vi "Acquisition & Generation (Init Memory) test.vi"   [LabVIEW 2014]
uses:
  <vilib>/Platform/TimedLoop/XDataNode/timing_clust.ctl
  <vilib>/Platform/TimedLoop/XDataNode/nitl_modes.ctl
  <vilib>/Platform/TimedLoop/XDataNode/wakeup.ctl
  <vilib>/rvi/Emulation/niFpgaSctlEmulationGetInTimedLoop.vi
  <vilib>/rvi/Emulation/niFpgaEmulationReportErrorSimple.vi
  <vilib>/rvi/Emulation/niFpgaGetClockAttributes.vi
  <vilib>/rvi/Emulation/niFpgaCriticalErrorInLSC.vi
  <vilib>/rvi/Memory/Memory_Emulation/nirvimemoryFastEmulation.vi
  <vilib>/rvi/Memory/Memory_Emulation/nirvimemoryEmulation.vi
  <vilib>/rvi/Emulation/niFpgaEmulationIsFPGAContextNoSignature.vi
  <vilib>/rvi/DataTransferAndStorage/Container/Common/niFpgaContainerGetUniqueNameForEmu.vi
  <vilib>/rvi/Emulation/niFpgaProcessEmulError.vi
  <vilib>/rvi/errors/nirviReportUnexpectedCaseInternalError (U32).vi
  <vilib>/rvi/errors/niFpgaSetErrorForExecOnDevCompSimple.vi
  <vilib>/rvi/eio/common/nirviEmuReportErrorAndStop.vi
  <vilib>/rvi/FIFO/Fifo_Resource/nirvififoEmulationSetSize.vi
  <vilib>/rvi/FIFO/Fifo_Resource/nirviFifoEmulationQueueMgr.vi
  <instcachedir>/0/nirviFifoEmulationQueueMgr_E5CAEC123FF24DC58D834DCA3CDAA9B5.lvgen/nirviFifoEmulationQueueMgr_E5CAEC123FF24DC58D834DCA3CDAA9B5_010.vi
  <vilib>/rvi/FIFO/Fifo_Resource/nirvififoEmulationDetermineInputValidOut.vi
  <vilib>/rvi/FIFO/Fifo_Resource/nirvififoEmulationCreateLock.vi
  <vilib>/rvi/FIFO/Fifo_Resource/nirvififoEmulationObtainLock.vi
  <vilib>/rvi/FIFO/Fifo_Resource/nirvififoEmulationReleaseLock.vi
  <vilib>/rvi/occurrence/nirviWaitOnOccurrenceBase.vi
  <vilib>/rvi/errors/nirviReportUnexpectedCaseInternalError.vi
  <vilib>/rvi/interface/RandomDataEmulation/niFpgaRandomDataHandleErrors.vi
  <vilib>/rvi/eio/common/nirviEmuTemplateMethod_errors.vi
  <vilib>/Platform/TimedLoop/XDataNode/XDataNode.xnode
  <vilib>/rvi/DataTransferAndStorage/Container/XNode/niFpgaContainer.xnode
  <vilib>/rvi/FIFO/Fifo_Resource/nirvififoEmulationWrite.vi
  <vilib>/rvi/interface/RandomDataEmulation/nirviRandomDataFpgaReadWriteTemplate.vi
  <vilib>/rvi/FIFO/Fifo_Resource/nirvififoEmulationRead.vi
  <vilib>/eio/EIOMethodNode/EIOMethodNode.xnode
  <vilib>/Platform/TimedLoop/XDataNode/XDNodeRunTimeDep.lvlib
types:
  T1 = typedef "XDNodeRunTimeDep.lvlib/timing_clust.ctl" = cluster{"Expected End [f-1]":u64, "Actual End [f-1]":u64, "Finished Late? [f-1]":bool, "Expected End [i-1]":u64, "Actual End [i-1]":u64, "Finished Late? [i-1]":bool, "Expected Start [i]":u64, "Actual Start [i]":u64, "Expected Start [f]":u64, "Actual Start [f]":u64, "Source Name":string, "Structure Name":string, "Period":i64, "Deadline":i64, "Offset":i64, "Start":i64, "Priority":i32, "Timeout":i32, "Mode":T2, "Wakeup Reason":T3, "Error":errorcluster, "Source Type":string, "Secondary Source Type":string, "Global End Time":u64, "Global Start Time":u64, "Frame Duration":u64, "Iteration Duration":u64, "Assigned CPU":i32, "I/O Scan Engine Mode":u32}
  T2 = typedef "XDNodeRunTimeDep.lvlib/nitl_modes.ctl" = enum32{"No Change", "Process missed periods, maintain original phase", "Discard missed periods, maintain original phase", "Process missed periods, ignore original phase", "Discard missed periods, ignore original phase"}
  T3 = typedef "XDNodeRunTimeDep.lvlib/wakeup.ctl" = enum32{"Normal", "Aborted", "Asynchronous wakeup", "Timing source error", "Timed loop error", "Timeout"}
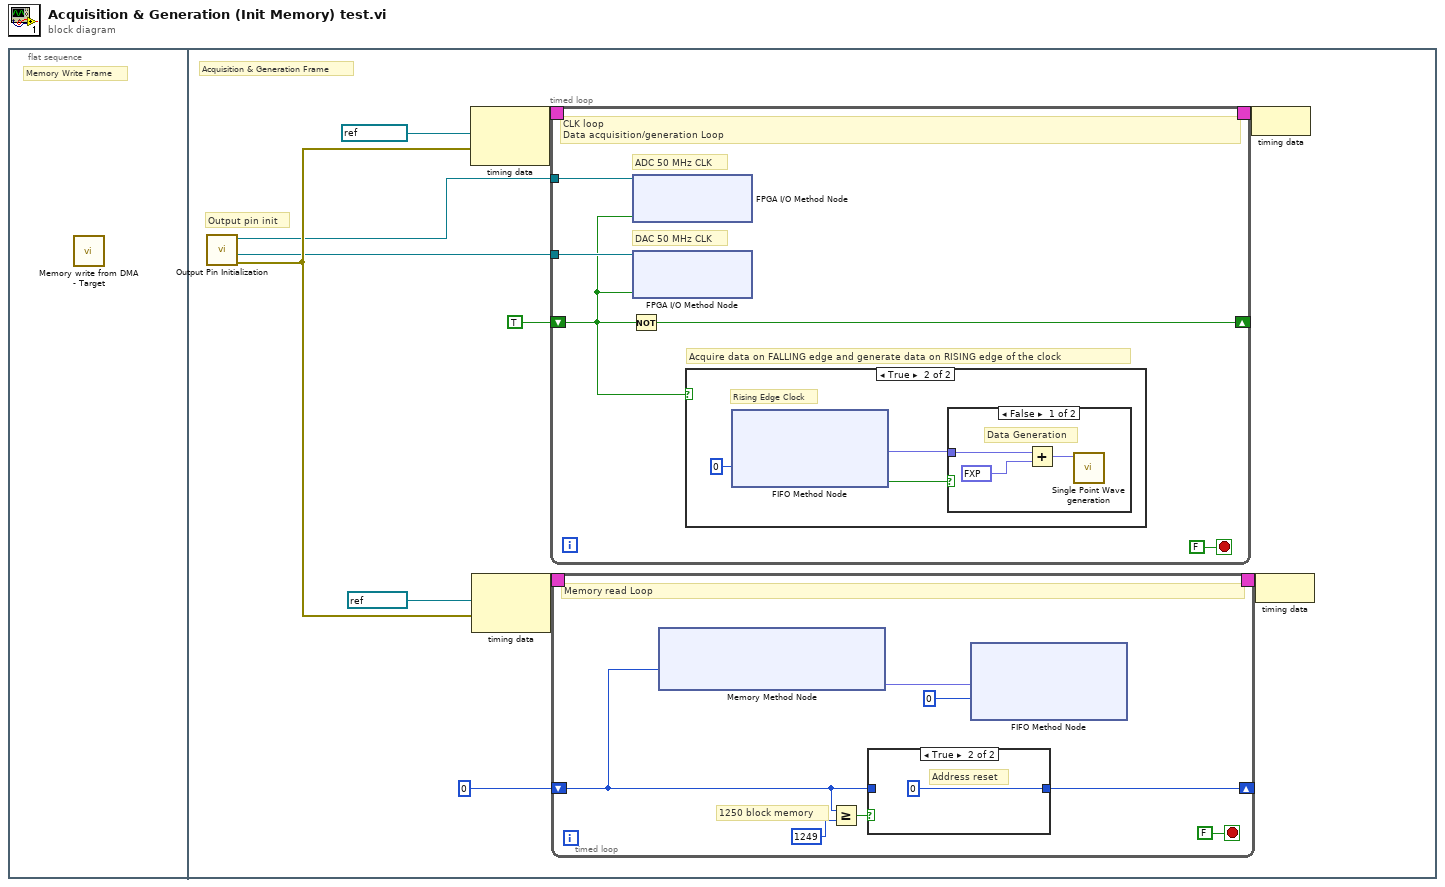
[diagram p0: block diagram]
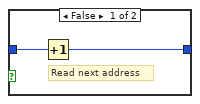
[diagram p2: hidden frame]
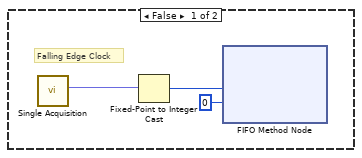
[diagram p3: hidden frame]
diagram:
  n1 = flat-sequence {
    frame #0 {
      # "Memory Write Frame"
      n2 = call "Memory write from DMA - Target.vi"() -> ()  [unwired: 12 in]
    }
    frame #1 {
      # "Acquisition & Generation Frame"
      # "Output pin init"
      n3 = call "Output Pin Initialization.vi"() -> ("error out"=w3:errorcluster, "I/O Out Clock DAC (pin16)"=w1:refnum<k21>, "I/O Out Clock ADC (pin17)"=w2:refnum<k21>)  [unwired: 8 in]
      n4 = node-c288(refnum<k21> "100MHz" ("Source Name"), w3) -> (w11:T1)
      n5 = node-c288(refnum<k21> "50MHz" ("Source Name"), w3) -> (w9:T1)
      n6 = timed-loop {
        timing: w11 -> [_]
        timing-out: [_] -> w10
        shift-right: [w31] -> _
        shift-left: TRUE -> [w29]
        tunnel: w2 -> [w33]
        tunnel: w1 -> [w30]
        stop <- FALSE stop-if-true
        # "DAC 50 MHz CLK"
        # "Acquire data on FALLING edge and generate data on RISING edge of the clock"
        # "ADC 50 MHz CLK"
        # "CLK loop\nData acquisition/generation Loop"
        n7 = Not(x=w29) -> (.not. x?=w31:bool)
        n8 = xnode "FPGA I/O Method Node"("FPGA I/O In"=w33, "Data"=w29) -> ()  [unwired: 1 out]
        n9 = xnode "FPGA I/O Method Node"("FPGA I/O In"=w30, "Data"=w29) -> ()  [unwired: 1 out]
        n10 = case shown="True" w29 {
          frame False {
            # "Falling Edge Clock"
            n11 = call "Single Acquisition.vi"() -> ("Out"=w34:fxp<+/-,12,12>)  [unwired: 10 in, 1 out]
            n12 = Fixed-Point to Integer Cast(1:w34) -> (0:w35:i16)
            n13 = xnode ("FIFO Method Node")("Element"=w35, "Timeout"=0) -> ()  [unwired: 1 in, 2 out]
          }
          frame True {
            # "Rising Edge Clock"
            n14 = xnode ("FIFO Method Node")("Timeout"=0) -> ("Element"=w37:fxp<+/-,12,12>, "Timed Out?"=w38:bool)  [unwired: 1 in, 1 out]
            n15 = case shown="False" w38 {
              tunnel: w37 -> [w42 _]
              frame False {
                # "Data Generation"
                n16 = Add(x=w42, y=fxp<+,12,12> 2048.0) -> (x+y=w40:fxp<+/-,14,14>)
                n17 = call "Single Point Wave generation.vi"("Data To Write"=w40) -> ()  [unwired: 10 in, 1 out]
              }
              frame True {
                # "FPGA memory slow"
              }
            }
          }
        }
      }
      n18 = timed-loop {
        timing: w9 -> [_]
        timing-out: [_] -> w8
        shift-right: [w16] -> _
        shift-left: u32 0 -> [w14]
        stop <- FALSE stop-if-true
        # "1250 block memory"
        # "Memory read Loop"
        n19 = xnode ("Memory Method Node")("Address"=w14) -> ("Data"=w13:fxp<+/-,12,12>)  [unwired: 1 in, 1 out]
        n20 = Greater Or Equal?(x=w14, y=u32 1249) -> (x >= y?=w17:bool)
        n21 = case shown="True" w17 {
          tunnel: w14 -> [w20 _]
          tunnel: [w19 u32 0] -> w16
          frame False {
            # "Read next address"
            n22 = Increment(x=w20) -> (x+1=w19:u32)
          }
          frame True {
            # "Address reset"
          }
        }
        n23 = xnode ("FIFO Method Node")("Element"=w13, "Timeout"=0) -> ()  [unwired: 1 in, 2 out]
      }
      n24 = node-c288(w10) -> ()
      n25 = node-c288(w8) -> ()
    }
  }
